vi "Tester-FPGA-Main.vi"() -> ()   [LabVIEW 2024]
uses:
  <vilib>/Platform/TimedLoop/XDataNode/wakeup.ctl
  <vilib>/Platform/TimedLoop/XDataNode/XDNodeRunTimeDep.lvlib
  <vilib>/Platform/TimedLoop/XDataNode/nitl_modes.ctl
  <vilib>/Platform/TimedLoop/XDataNode/timing_clust.ctl
  <vilib>/Platform/TimedLoop/XDataNode/XDataNode.xnode
  <vilib>/eio/EIONode/EIONode.xnode
  <vilib>/rvi/eio/common/nirviEmuTemplateMethod_errors.vi
panel:
  out "ReadVoltageOut":i16
  out "ReadDO2":bool
  out "ReadDO1":bool
  in  "STOP FPGA":bool
  out "Measured Period (Ticks)":u32
  out "Low Period (Ticks)":u32
  out "High Period (Ticks)":u32
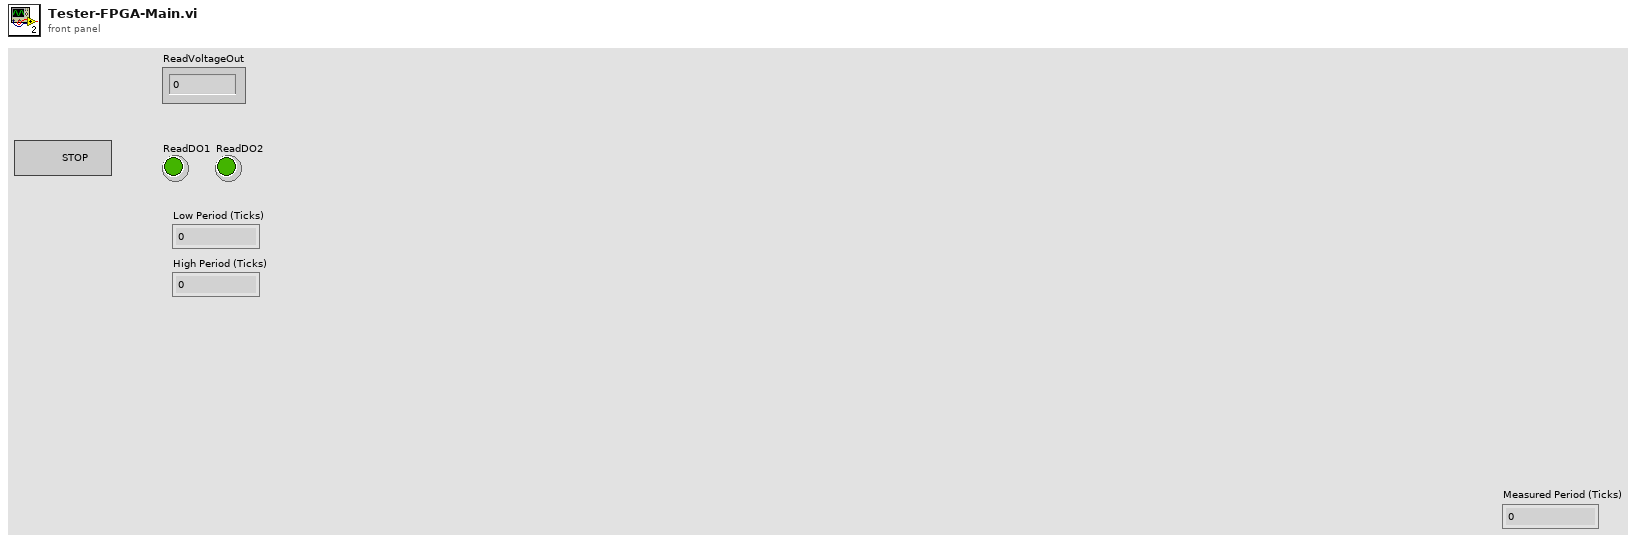
[diagram p1: front panel]
types:
  T1 = typedef "XDNodeRunTimeDep.lvlib/timing_clust.ctl" = cluster{"Expected End [f-1]":u64, "Actual End [f-1]":u64, "Finished Late? [f-1]":bool, "Expected End [i-1]":u64, "Actual End [i-1]":u64, "Finished Late? [i-1]":bool, "Expected Start [i]":u64, "Actual Start [i]":u64, "Expected Start [f]":u64, "Actual Start [f]":u64, "Source Name":string, "Structure Name":string, "Period":i64, "Deadline":i64, "Offset":i64, "Start":i64, "Priority":i32, "Timeout":i32, "Mode":T2, "Wakeup Reason":T3, "Error":errorcluster, "Source Type":string, "Secondary Source Type":string, "Global End Time":u64, "Global Start Time":u64, "Frame Duration":u64, "Iteration Duration":u64, "Assigned CPU":i32, "I/O Scan Engine Mode":u32}
  T2 = typedef "XDNodeRunTimeDep.lvlib/nitl_modes.ctl" = enum32{"No Change", "Process missed periods, maintain original phase", "Discard missed periods, maintain original phase", "Process missed periods, ignore original phase", "Discard missed periods, ignore original phase"}
  T3 = typedef "XDNodeRunTimeDep.lvlib/wakeup.ctl" = enum32{"Normal", "Aborted", "Asynchronous wakeup", "Timing source error", "Timed loop error", "Timeout"}
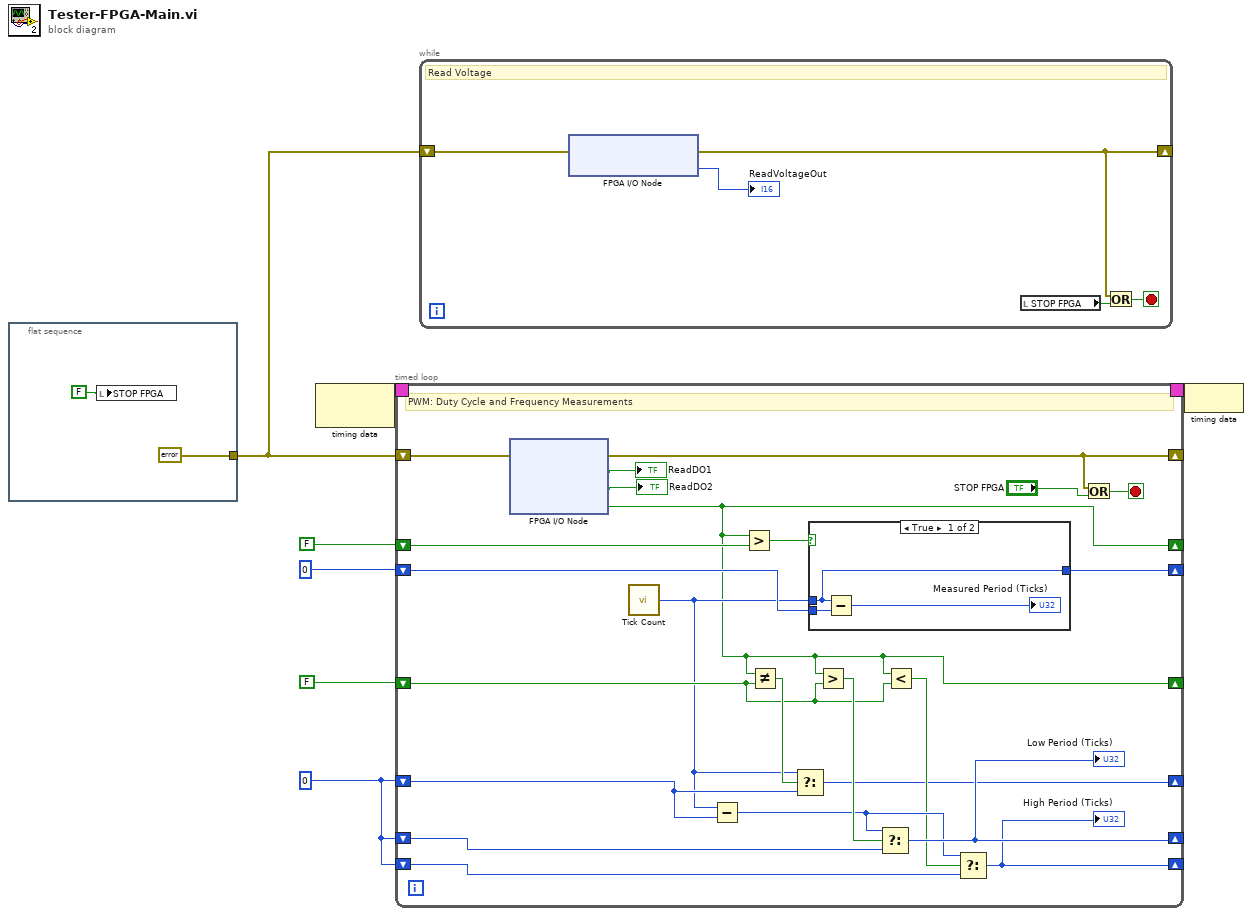
[diagram p0: block diagram]
diagram:
  w2 = u32 0 ("Tick Count(Ticks)")
  n1 = flat-sequence {
    tunnel: [errorcluster {"status"=FALSE, "code"=0, "source"=""} ("error out")] -> w1
    frame #0 {
      n2 = local write "STOP FPGA"(FALSE ("STOP FPGA")) -> ()
    }
  }
  n3 = node-c288() -> (w7:T1)  [unwired: 1 in]
  n4 = timed-loop {
    shift-left: w2 -> [w23]
    shift-right: [w24] -> _
    shift-left: w2 -> [w29]
    shift-right: [w30] -> _
    shift-left: FALSE ("Input") -> [w26]
    shift-right: [w13] -> _
    shift-left: w2 -> [w31]
    shift-right: [w22] -> _
    timing: w7 -> [_]
    timing-out: [_] -> w6
    shift-right: [w13] -> _
    shift-left: FALSE ("Digital Signal A") -> [w21]
    shift-right: [w19] -> _
    shift-left: u32 0 ("Tick Count(Ticks)") -> [w20]
    shift-right: [w14] -> _
    shift-left: w1 -> [w16]
    stop <- w15 stop-if-true
    # "PWM: Duty Cycle and Frequency Measurements"
    n5 = xnode "FPGA I/O Node"("error in"=w16) -> ("error out"=w14:errorcluster, "ReadDO1"=→"ReadDO1":bool, "ReadDO2"=→"ReadDO2":bool, "ReadPWM"=w13:bool)  [unwired: 3 in, 3 out]
    n6 = call "Tick Count"() -> ("Tick Count(Ticks)"=w17:u32)
    n7 = Subtract(x=w17, y=w31) -> (x-y=w27:u32)
    n8 = Greater?(x=w13, y=w21) -> (0:w18:bool)
    n9 = Not Equal?(x=w13, y=w26) -> (x != y?=w32:bool)
    n10 = Select(t=w17, s=w32, f=w31) -> (s? t:f=w22:u32)
    n11 = case shown="True" w18 {
      tunnel: w17 -> [w33 _]
      tunnel: w20 -> [w34 w36]
      tunnel: [w33 w36] -> w19
      frame True {
        n12 = Subtract(x=w33, y=w34) -> (x-y=→"Measured Period (Ticks)":u32)
      }
      frame False {
      }
    }
    n13 = Greater?(x=w13, y=w26) -> (0:w28:bool)
    n14 = Select(t=w27, s=w28, f=w29) -> (s? t:f=w30:u32)
    "Low Period (Ticks)" <- w30
    n15 = Less?(x=w13, y=w26) -> (x < y?=w25:bool)
    n16 = Select(t=w27, s=w25, f=w23) -> (s? t:f=w24:u32)
    "High Period (Ticks)" <- w24
    n17 = Or(x=w14, y="STOP FPGA") -> (x .or. y?=w15:bool)
  }
  n18 = while {
    shift-right: [w39] -> _
    shift-left: w1 -> [w43]
    stop <- w40 stop-if-true
    # "Read Voltage"
    n19 = xnode "FPGA I/O Node"("error in"=w43) -> ("error out"=w39:errorcluster, "ReadVoltageOut"=→"ReadVoltageOut":i16)  [unwired: 1 in, 1 out]
    n20 = local read "STOP FPGA"() -> (w41:bool)
    n21 = Or(x=w39, y=w41) -> (x .or. y?=w40:bool)
  }
  n22 = node-c288(w6) -> ()
